vi "ReadPolarzationFile.vi"(1 "本次文件名":string) -> ()   [LabVIEW 2018]
uses:
  Init/AllPath.vi
  <vilib>/Utility/file.llb/Read Delimited Spreadsheet (string).vi
  HistoryFile.vi
panel:
  out "偏振方向":string
  out "偏振度":string
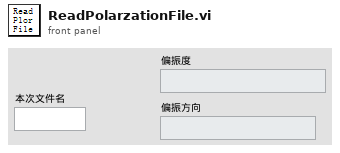
[diagram p1: front panel]
types:
  T1 = cluster{"能量/功率":path, " 示波器":path, " 光谱仪":path, "偏振":path, "近远场":cluster{" 近场图片":path, " 远场图片":path, "发散角数据":path}, "参数":path, " 基路径":path, "文件名信息":path, "输出模板路径":path, "输出报告路径":path, "位置信息路径":path}
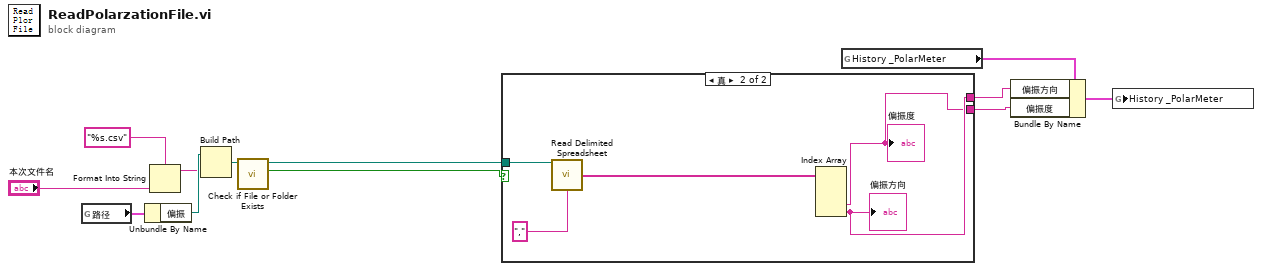
[diagram p0: block diagram]
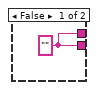
[diagram p2: hidden frame]
diagram:
  n1 = global read "AllPath.vi" "路径"() -> (w12:T1)
  n2 = Unbundle By Name(w12) -> ("偏振"=w11:path)
  n3 = Format Into String(format string="%s.csv" ("格式字符串"), "本次文件名") -> (resulting string=w8:string)  [unwired: 2 in, 1 out]
  n4 = Build Path(base path=w11, name or relative path=w8) -> (appended path=w7:path)
  n5 = call <vilib>:"Check if File or Folder Exists.vi"("path"=w7) -> ("file or folder exists?"=w6:bool, "dup path"=w5:path)  [unwired: 8 in, 1 out]
  n6 = case shown="真" w6 {
    tunnel: w5 -> [_ w16]
    tunnel: [w13 w15] -> w4
    tunnel: [w13 w14] -> w3
    frame False {
      w13 = ""
    }
    frame True {
      n7 = call-poly <vilib>:"Read Delimited Spreadsheet.vi"("file path (dialog if empty)"=w16, "delimiter (\\t)"="," ("delimiter (\\t)")) -> ("first row"=w18:string[])  [unwired: 8 in, 5 out]
      n8 = Index Array(array=w18) -> (element #3=w14:string, element #4=w15:string)  [unwired: 4 in, 2 out]
      "偏振度" <- w14
      "偏振方向" <- w15
    }
  }
  n9 = global read "HistoryFile.vi" "History _PolarMeter"() -> (w2:cluster{" 偏振方向":string, "偏振度":string})
  n10 = Bundle By Name(cluster=w2, "偏振方向"=w4, "偏振度"=w3) -> (w1:cluster{" 偏振方向":string, "偏振度":string})
  n11 = global write "HistoryFile.vi" "History _PolarMeter"(w1) -> ()
